vi "Get XML Node Context.vi"() -> ()   [LabVIEW 2018]
panel:
  in  "Node Name":string
  in  "error in (no error)":errorcluster
  in  "File Contents":string
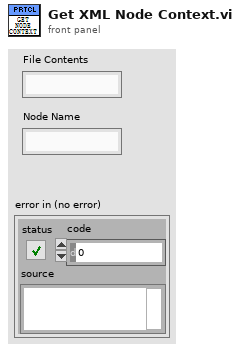
[diagram p1: front panel]
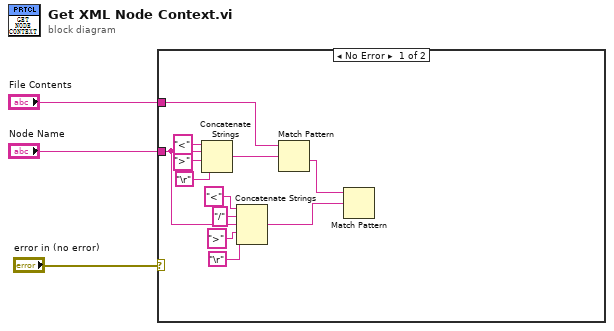
[diagram p0: block diagram]
diagram:
  n1 = case shown="No Error" "error in (no error)" {
    tunnel: "File Contents" -> [w12 _]
    tunnel: "Node Name" -> [w10 _]
    frame No Error {
      n2 = Concatenate Strings("<" ("string"), w10, ">" ("string"), "\r") -> (w11:string)
      n3 = Concatenate Strings("<" ("string"), "/" ("string"), w10, ">" ("string"), "\r") -> (w4:string)
      n4 = Match Pattern(string=w12, regular expression=w11) -> (after substring=w5:string)  [unwired: 1 in, 3 out]
      n5 = Match Pattern(string=w5, regular expression=w4) -> ()  [unwired: 1 in, 4 out]
    }
    frame Error {
    }
  }
